vi "Add to Inventory.vi"() -> ()   [LabVIEW 2013]
uses:
  Controls/Add Component Line.ctl
  Controls/Components.ctl
  Controls/Component Sub Type.ctl
  Globals/Inventory Path Global.vi
  <vilib>/Utility/file.llb/Write To Spreadsheet File (string).vi
panel:
  in  "Add":bool
  in  "Add Component Line":T1
  # "Add to Home Lab. Inventory"
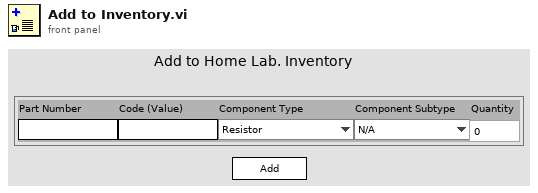
[diagram p1: front panel]
types:
  T1 = typedef "Add Component Line.ctl" = cluster{"Part Number":string, "Code (Value)":string, "Component Type":T2, "Component Subtype":T3, "Quantity":u32}
  T2 = typedef "Components.ctl" = enum16{"Resistor", "Capacitor", "Diode", "Voltage Regulator", "Transistors", "ICs"}
  T3 = typedef "Component Sub Type.ctl" = enum16{"N/A", "Carbon", "Variable - Trimmer", "Variable - Pot", "Ceramic", "Electrolitic", "Zenner", "TO-92", "TO-220", "NPN", "PNP", "CMOS", "Processor"}
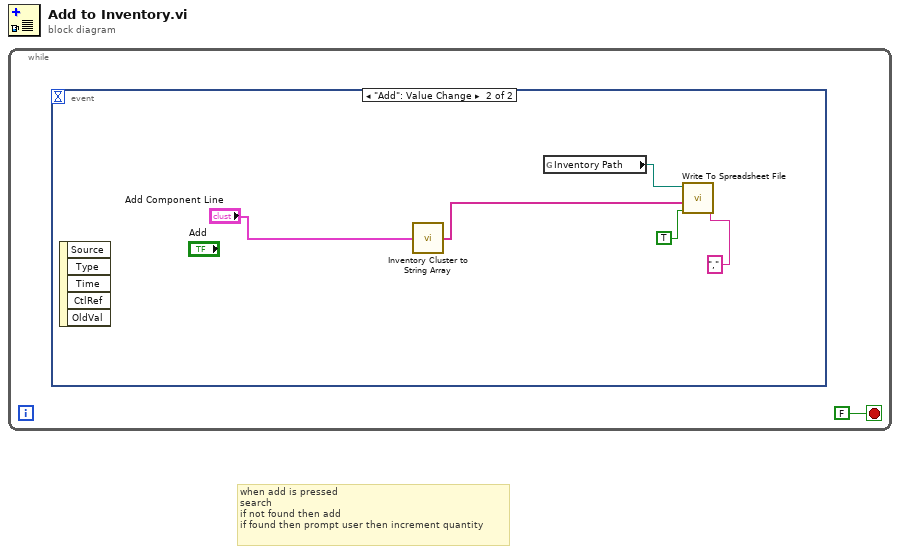
[diagram p0: block diagram]
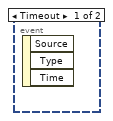
[diagram p2: hidden frame]
diagram:
  # "when add is pressed\nsearch\nif not found then add\nif found then prompt user then increment quantity"
  n1 = while {
    stop <- FALSE stop-if-true
    n2 = event shown="[1] \"Add\": Value Change" {
      selector: _ -> [_ _]
      dyn-events: _ -> [_ _]
      timeout: _ -> [_ _]
      event Timeout {
        n3 = event-data() -> ()  [unwired: 1 in, 3 out]
      }
      event "Add": Value Change {
        n4 = event-data() -> ()  [unwired: 1 in, 5 out]
        n5 = call "Inventory Cluster to String Array.vi"("Component Line"="Add Component Line") -> ("Array"=w6:string[])
        n6 = global read "Inventory Path Global.vi" "Inventory Path"() -> (w4:path)
        n7 = call-poly <vilib>:"Write To Spreadsheet File.vi"("delimiter (\\t)"="," ("delimiter (\\t)"), "append to file? (new file:F)"=TRUE, "1D data"=w6, "file path (dialog if empty)"=w4) -> ()  [unwired: 4 in, 1 out]
      }
    }
  }
